vi "Actor Core.vi"(8 "error in":errorcluster, 11 "Timed Loop Controller in":refnum<class "Timed Loop Controller.lvclass">) -> (0 "error out":errorcluster, 3 "Actor out":refnum<class "Actor.lvclass">)   [LabVIEW 2012, in "Timed Loop Controller.lvlib" / "Timed Loop Controller.lvclass"]
doc: "(<B>Filename</B>: Actor Framework.lvlib:Actor.lvclass:Actor Core.vi)\n\nReceives messages to the actor, reacts to them, and initiates any error handling that may shut the actor down.\n\nDescendant classes may override this VI to append parallel tasks for the actor to complete while it handles messages. Overrides use the Call Parent Method node."
uses:
  Timed Loop Controller.lvclass
  <vilib>/ActorFramework/Actor/Actor.lvclass
  <vilib>/ActorFramework/Actor/Actor.lvclass/Actor.ctl
  <vilib>/ActorFramework/Message Enqueuer/Message Enqueuer.lvclass/Message Enqueuer.ctl
  Timed Loop Controller.lvclass/Timed Loop Controller.ctl
  <vilib>/ActorFramework/Message Enqueuer/Init from Existing Queue.vi
  <vilib>/ActorFramework/Message Enqueuer/Enqueue.vi
  <vilib>/ActorFramework/Message Priority Queue/Priority Enqueue.vi
  <vilib>/ActorFramework/Message Enqueuer/Message Enqueuer.lvclass
  Timed Loop Controller Messages/Update Msg/Update Msg.lvclass
panel:
  in  "Stop?":bool
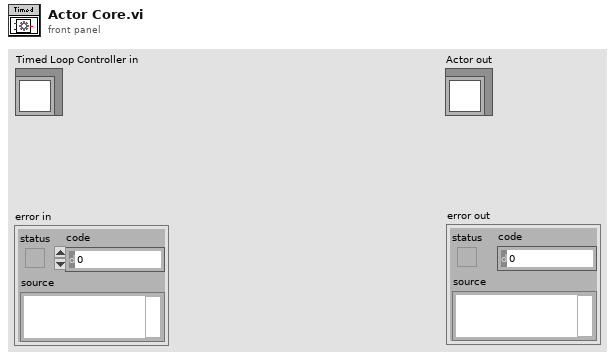
[diagram p1: front panel]
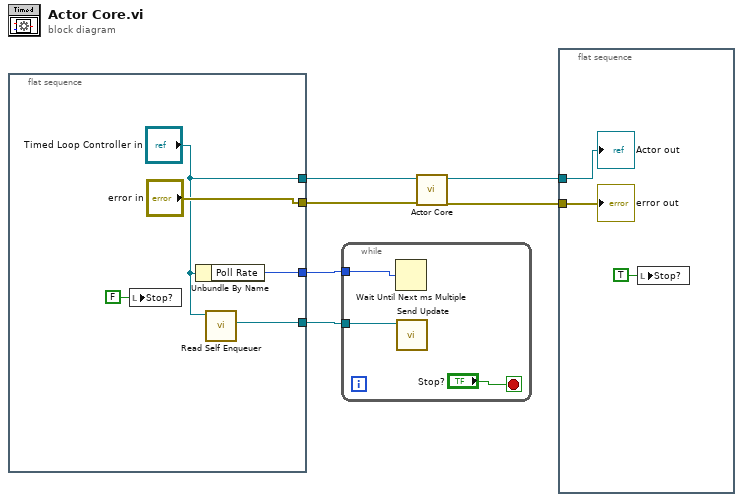
[diagram p0: block diagram]
diagram:
  n1 = flat-sequence {
    tunnel: ["error in"] -> w4
    tunnel: ["Timed Loop Controller in"] -> w3
    tunnel: [w9] -> w2
    tunnel: [w8] -> w1
    frame #0 {
      n2 = local write "Stop?"(FALSE ("Stop?")) -> ()
      n3 = Unbundle By Name("Timed Loop Controller in") -> ("Poll Rate"=w9:i64)
      n4 = call <vilib>:"Read Self Enqueuer.vi"("Actor"="Timed Loop Controller in") -> ("Self Enqueuer"=w8:refnum<class "Message Enqueuer.lvclass">)  [unwired: 10 in]
    }
  }
  n5 = while {
    tunnel: w2 -> [w13]
    tunnel: w1 -> [w12]
    stop <- "Stop?" stop-if-true
    n6 = Wait Until Next ms Multiple(millisecond multiple=w13) -> ()  [unwired: 1 out]
    n7 = call "Send Update.vi"("Message Enqueuer"=w12) -> ()  [unwired: 9 in, 2 out]
  }
  n8 = call-parent "Actor Core.vi"("error in"=w4, "Actor in"=w3) -> ("error out"=w6:errorcluster, "Actor out"=w5:refnum<class "Actor.lvclass">)  [unwired: 8 in]
  n9 = flat-sequence {
    tunnel: w6 -> [w17]
    tunnel: w5 -> [w16]
    frame #0 {
      n10 = local write "Stop?"(TRUE ("Stop?")) -> ()
      "error out" <- w17
      "Actor out" <- w16
    }
  }
